vi "Recurse Maze.vi"(7 "Visit only once?":bool, 8 "error in (no error)":errorcluster, 10 "Current Cell":T1, 11 "Maze In":refnum<class "Maze.lvclass">) -> (0 "error out":errorcluster, 1 "Step Count":i32, 2 "Steps":cluster{"row":i32, "col":i32}[](array[cluster]), 3 "Maze Out":refnum<class "Maze.lvclass">)   [LabVIEW 2021, in "Maze.lvclass"]
uses:
  Maze.lvclass
  Maze.lvclass/Maze.ctl
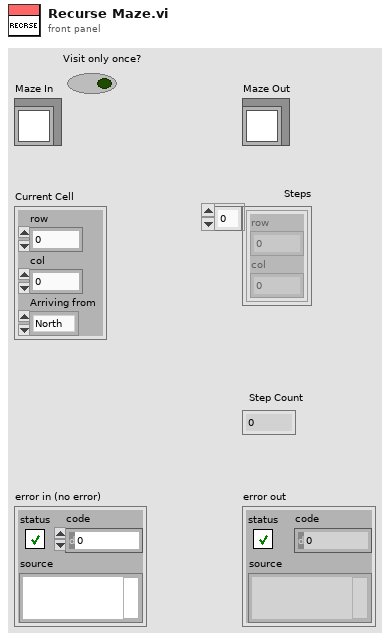
[diagram p1: front panel]
types:
  T1 = cluster{"row":i32, "col":i32, "Arriving from":enum16{"North", "South", "East", "West"}}
  T2 = cluster{"row":i32, "col":i32, "Arriving from":enum16{"North", "South", "East", "West"}}[]
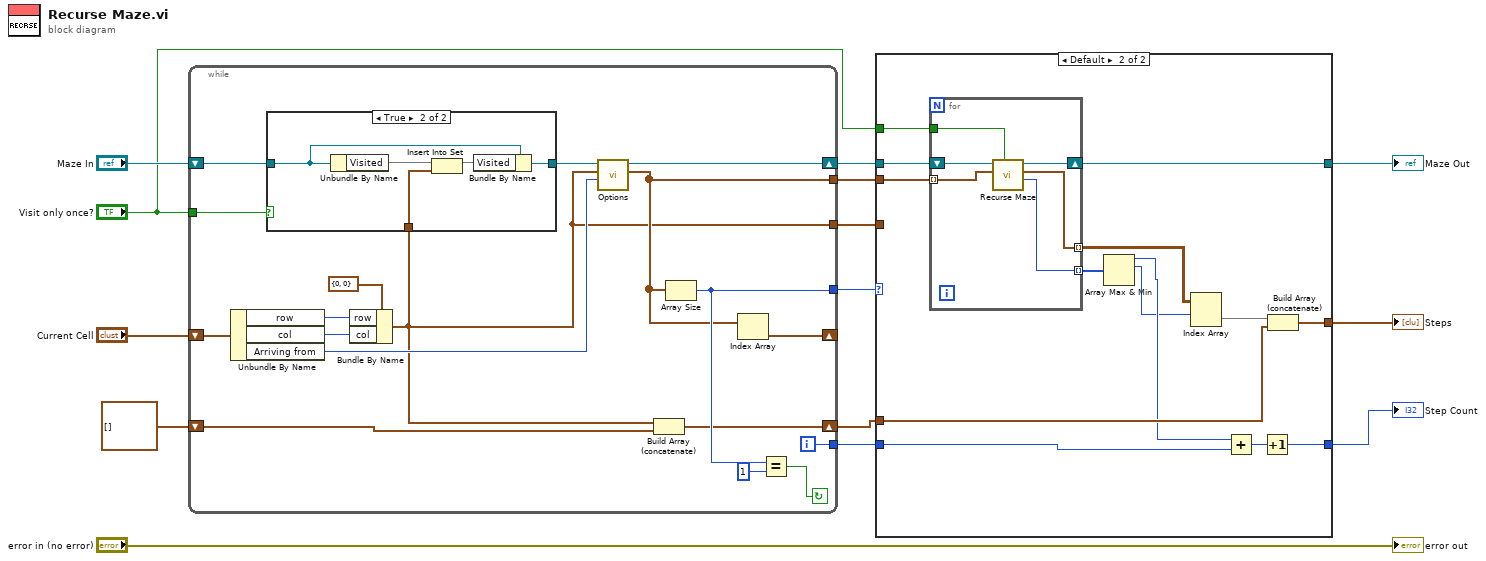
[diagram p0: block diagram]
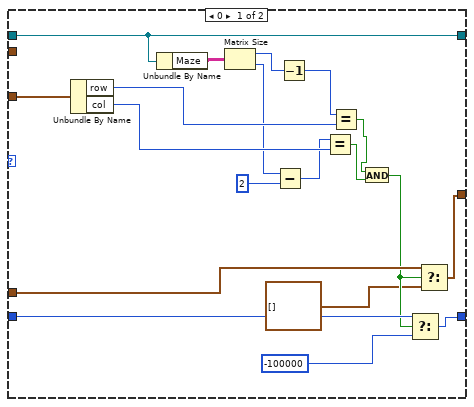
[diagram p3: hidden frame]
diagram:
  n1 = while {
    tunnel: [w31] -> w8
    shift-right: [w32] -> w9
    shift-left: "Maze In" -> [w18]
    tunnel: [w28] -> w7
    shift-right: [w21] -> _
    shift-left: "Current Cell" -> [w24]
    tunnel: [w22] -> w5
    shift-right: [w20] -> w6
    shift-left: cluster{"row":i32, "col":i32}[] [] ("output cluster") -> [w19]
    tunnel: "Visit only once?" -> [w16]
    tunnel: [w15] -> w3
    i -> [w28]
    stop <- w29 continue-if-true
    n2 = Unbundle By Name(w24) -> ("row"=w25:i32, "col"=w26:i32, "Arriving from"=w23:enum16{"North", "South", "East", "West"})
    n3 = Bundle By Name(cluster=cluster{"row":i32, "col":i32} {"row"=0, "col"=0} ("Cluster"), "row"=w25, "col"=w26) -> (w15:cluster{"row":i32, "col":i32})
    n4 = case shown="True" w16 {
      tunnel: w18 -> [w33 w38]
      tunnel: [w33 w37] -> w17
      tunnel: w15 -> [_ w36]
      frame False {
      }
      frame True {
        n5 = Unbundle By Name(w38) -> ("Visited"=w34:set{cluster{"row":i32, "col":i32}})
        n6 = Insert Into Set(10:w36, 11:w34) -> (3:w35:set{cluster{"row":i32, "col":i32}})  [unwired: 1 out]
        n7 = Bundle By Name(cluster=w38, "Visited"=w35) -> (w37:refnum<class "Maze.lvclass">)
      }
    }
    n8 = call "Options.vi"("Arriving from"=w23, "Cluster"=w15, "Maze In"=w17) -> ("Possible Steps"=w22:T2, "Maze Out"=w32:refnum<class "Maze.lvclass">)  [unwired: 6 in, 1 out]
    n9 = Build Array (concatenate)(w15, w19) -> (w20:cluster{"row":i32, "col":i32}[])
    n10 = Array Size(array=w22) -> (size(s)=w31:i32)
    n11 = Index Array(array=w22) -> (element=w21:T1)  [unwired: 1 in]
    n12 = Equal?(x=w31, y=1) -> (x = y?=w29:bool)
  }
  n13 = case shown="Default" w8 {
    tunnel: [w54 w71] -> w13
    tunnel: [w46 w68] -> w12
    tunnel: [w41 w70] -> w11
    tunnel: w9 -> [w54 w69]
    tunnel: w6 -> [w56 w66]
    tunnel: w5 -> [_ w65]
    tunnel: w7 -> [w57 w64]
    tunnel: w3 -> [w55 _]
    tunnel: "Visit only once?" -> [_ w63]
    frame 0 {
      n14 = Unbundle By Name(w55) -> ("row"=w49:i32, "col"=w48:i32)
      n15 = Unbundle By Name(w54) -> ("Maze"=w53:string[][])
      n16 = Matrix Size(0:w53) -> (1:w52:i32, 2:w45:i32)
      n17 = Subtract(x=w45, y=2) -> (x-y=w47:i32)
      n18 = Decrement(x=w52) -> (x-1=w51:i32)
      n19 = Equal?(x=w47, y=w48) -> (x = y?=w43:bool)
      n20 = Equal?(x=w51, y=w49) -> (x = y?=w44:bool)
      n21 = And(x=w44, y=w43) -> (x .and. y?=w40:bool)
      n22 = Select(t=w57, s=w40, f=-100000) -> (s? t:f=w46:i32)
      n23 = Select(t=w56, s=w40, f=cluster{"row":i32, "col":i32}[] []) -> (s? t:f=w41:cluster{"row":i32, "col":i32}[])
    }
    frame Default {
      n24 = for {
        shift-right: [w76] -> w71
        shift-left: w69 -> [w77]
        tunnel: w65 -> [w75] mode=indexing
        tunnel: [w74] -> w62 mode=indexing
        tunnel: [w73] -> w67 mode=indexing
        tunnel: w63 -> [w72]
        n25 = call "Recurse Maze.vi"("Visit only once?"=w72, "Current Cell"=w75, "Maze In"=w77) -> ("Step Count"=w74:i32, "Steps"=w73:cluster{"row":i32, "col":i32}[], "Maze Out"=w76:refnum<class "Maze.lvclass">)  [unwired: 5 in, 1 out]
      }
      n26 = Array Max & Min(array=w62) -> (max value=w59:i32, max index (indices)=w58:i32)  [unwired: 2 out]
      n27 = Index Array(array=w67, index (row)=w58) -> (element=w61:cluster{"row":i32, "col":i32}[])  [unwired: 1 in]
      n28 = Add(x=w59, y=w64) -> (x+y=w60:i32)
      n29 = Increment(x=w60) -> (x+1=w68:i32)
      n30 = Build Array (concatenate)(w61, w66) -> (w70:cluster{"row":i32, "col":i32}[])
    }
  }
  "Maze Out" <- w13
  "Step Count" <- w12
  "Steps" <- w11
  "error out" <- "error in (no error)"
